vi "Example Grey.vi"() -> ()   [LabVIEW 2020]
uses:
  <vilib>/Utility/sysdir.llb/System Directory Type.ctl
  Sources/_Helpers/Tiff Page Details.ctl
  <vilib>/Analysis/1siggen.llb/Ramp Pattern by Samples.vi
  Sources/TIFF Writer/TIFF Writer.lvclass
  Sources/LV Tiff.lvlib
  Sources/TIFF Reader/TIFF Reader.lvclass
  <vilib>/Analysis/NI_AALBase.lvlib
panel:
  out "DBL":dbl[][](graph)
  out "Read DBL":dbl[][](graph)
  out "U8":u8[][](graph)
  out "Read U8":u8[][](graph)
  out "Read U16":u16[][](graph)
  out "U16":u16[][](graph)
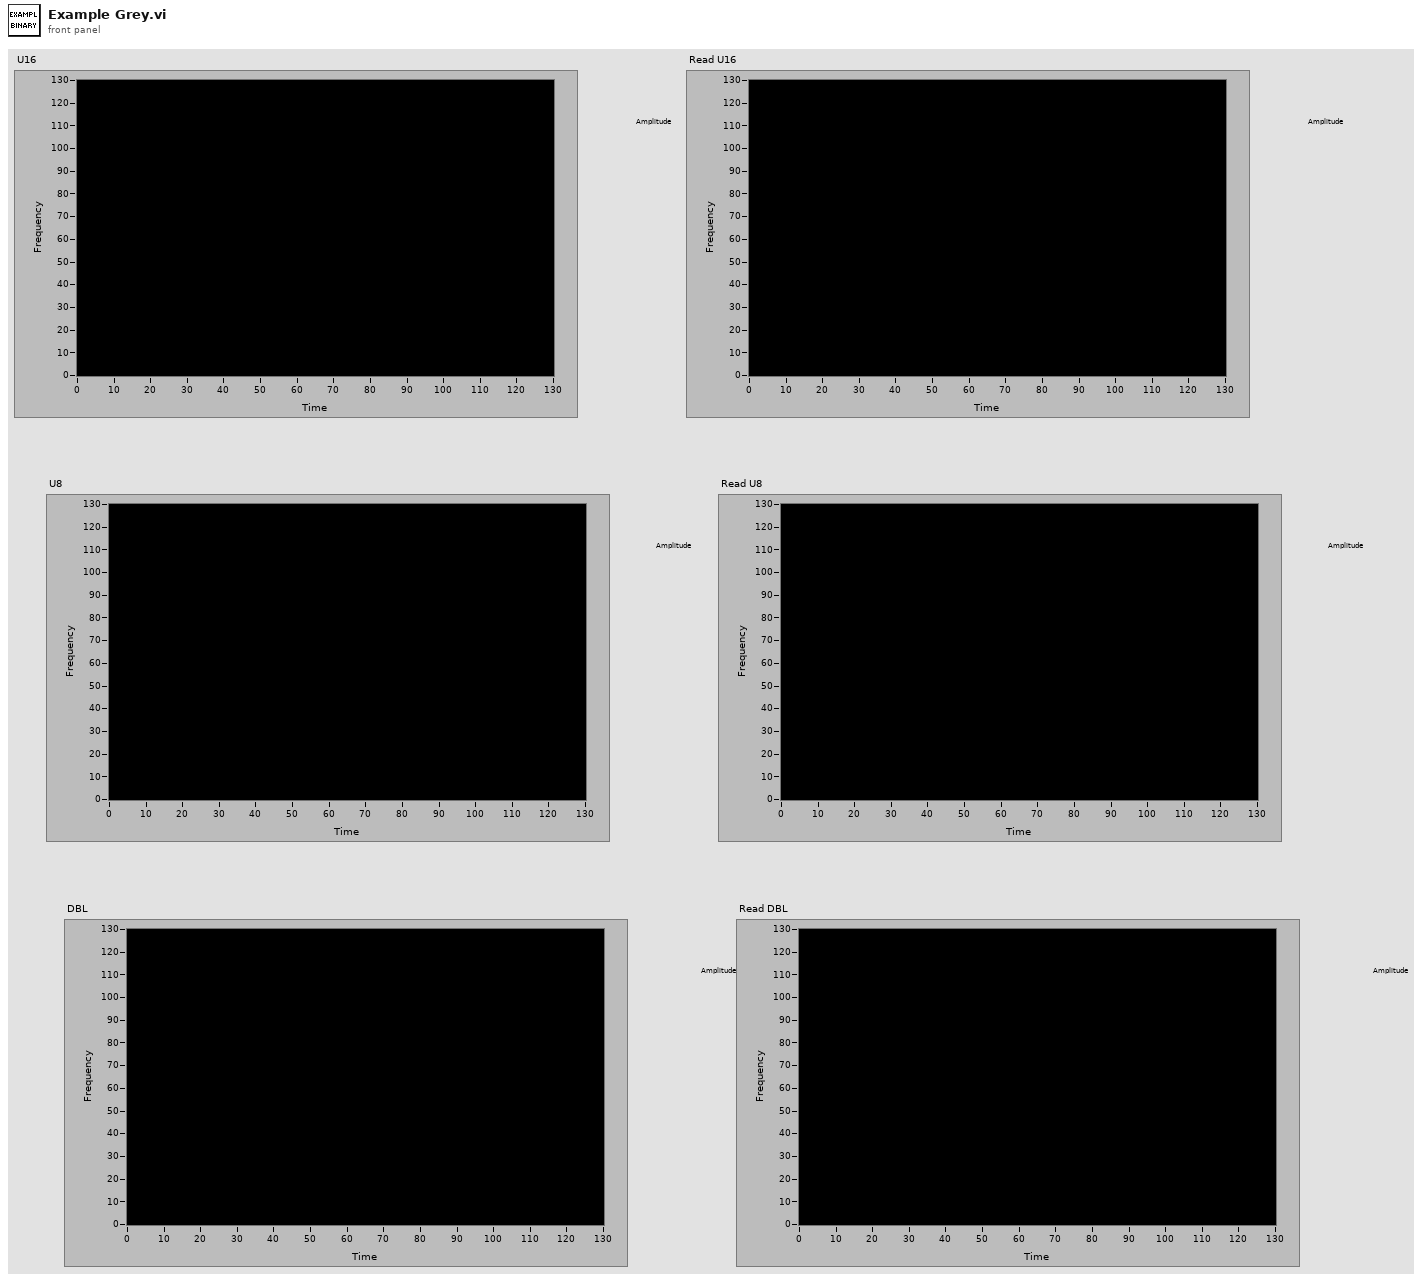
[diagram p1: front panel]
types:
  T1 = typedef "LV Tiff.lvlib/Tiff Page Details.ctl" = cluster{"ImageDescription":string, "XResolution":dbl, "YResolution":dbl, "ResolutionUnit":enum16{"None", "Inch", "Centimeter"}, "PhotometricInterpretation":u16, "Compression":enum16{"None", "Deflate", "JPEG"}, "PageName":string, "DocumentName":string}
  T2 = enum16{"open", "replace", "create", "open or create", "replace or create", "replace or create with confirmation"}
  T3 = typedef "System Directory Type.ctl" = i32
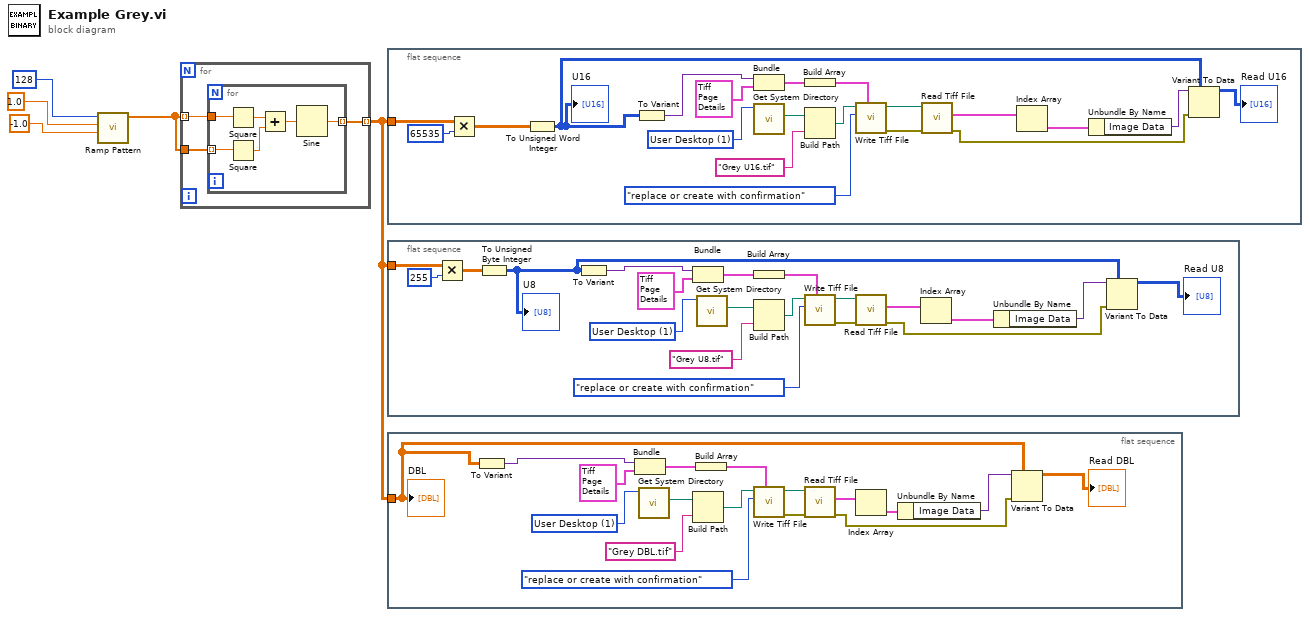
[diagram p0: block diagram]
diagram:
  n1 = call-poly <vilib>:"Ramp Pattern.vi"("start"=-1.0, "end"=1.0, "samples"=128) -> ("Ramp Pattern"=w2:dbl[])  [unwired: 7 in, 1 out]
  n2 = for {
    tunnel: [w8] -> w1 mode=indexing
    tunnel: w2 -> [w7] mode=indexing
    tunnel: w2 -> [w6]
    n3 = for {
      tunnel: [w14] -> w8 mode=indexing
      tunnel: w7 -> [w11]
      tunnel: w6 -> [w10] mode=indexing
      n4 = Square(x=w11) -> (x^2=w12:dbl)
      n5 = Square(x=w10) -> (x^2=w13:dbl)
      n6 = Add(x=w12, y=w13) -> (x+y=w9:dbl)
      n7 = Sine(x=w9) -> (sin(x)=w14:dbl)
    }
  }
  n8 = flat-sequence {
    tunnel: w1 -> [w20]
    frame #0 {
      w17 = T3 1 items=["User Home"=0, "User Desktop"=1, "User Documents"=2, "User Application Data"=3, "User Preferences"=4, "User Temporary"=5, "Public Documents"=6, "Public Application Data"=7, "Public Preferences"=8, "Public Cache"=13, "System Core Libraries"=9, "System Installed Libraries"=10, "Application Files"=11, "Boot Volume Root"=12] ("system directory type")
      n9 = Multiply(x=w20, y=u16 65535) -> (x*y=w33:dbl[][])
      n10 = To Unsigned Word Integer(number=w33) -> (unsigned 16bit integer=w34:u16[][])
      "U16" <- w34
      n11 = To Variant(anything=w34) -> (Variant=w24:variant)
      n12 = Bundle("Variant"=w24, "Details"=T1 {"ImageDescription"="", "XResolution"=0.0, "YResolution"=0.0, "ResolutionUnit"=enum."Inch", "PhotometricInterpretation"=34892, "Compression"=enum."None", "PageName"="", "DocumentName"=""}) -> (w25:cluster{"Variant":variant, "Details":T1})  [unwired: 1 in]
      n13 = call <vilib>:"Get System Directory.vi"("system directory type"=w17) -> ("system directory"=w22:path)  [unwired: 10 in]
      n14 = Build Array(w25) -> (w26:cluster{"Variant":variant, "Details":T1}[])
      n15 = Build Path(base path=w22, name or relative path="Grey U16.tif") -> (appended path=w23:path)
      n16 = call "Write Tiff File.vi"("Pages"=w26, "operation (replace)"=T2."replace or create with confirmation", "Path"=w23) -> ("error out"=w28:errorcluster, "path"=w27:path)  [unwired: 7 in]
      n17 = call "Read Tiff File.vi"("error in (no error)"=w28, "Path"=w27) -> ("error out"=w15:errorcluster, "Pages"=w29:cluster{"Image Data":variant, "Details":T1}[])  [unwired: 6 in, 2 out]
      n18 = Index Array(array=w29) -> (element=w30:cluster{"Image Data":variant, "Details":T1})  [unwired: 1 in]
      n19 = Unbundle By Name(w30) -> ("Image Data"=w31:variant)
      n20 = Variant To Data(error in=w15, type=w34, Variant=w31) -> (data=→"Read U16":u16[][])  [unwired: 1 out]
    }
  }
  n21 = flat-sequence {
    tunnel: w1 -> [w40]
    frame #0 {
      w37 = T3 1 items=["User Home"=0, "User Desktop"=1, "User Documents"=2, "User Application Data"=3, "User Preferences"=4, "User Temporary"=5, "Public Documents"=6, "Public Application Data"=7, "Public Preferences"=8, "Public Cache"=13, "System Core Libraries"=9, "System Installed Libraries"=10, "Application Files"=11, "Boot Volume Root"=12] ("system directory type")
      n22 = Multiply(x=w40, y=u8 255) -> (x*y=w53:dbl[][])
      n23 = To Unsigned Byte Integer(number=w53) -> (unsigned 8bit integer=w54:u8[][])
      "U8" <- w54
      n24 = To Variant(anything=w54) -> (Variant=w44:variant)
      n25 = Bundle("Variant"=w44, "Details"=T1 {"ImageDescription"="", "XResolution"=0.0, "YResolution"=0.0, "ResolutionUnit"=enum."Inch", "PhotometricInterpretation"=34892, "Compression"=enum."None", "PageName"="", "DocumentName"=""}) -> (w45:cluster{"Variant":variant, "Details":T1})  [unwired: 1 in]
      n26 = call <vilib>:"Get System Directory.vi"("system directory type"=w37) -> ("system directory"=w42:path)  [unwired: 10 in]
      n27 = Build Array(w45) -> (w46:cluster{"Variant":variant, "Details":T1}[])
      n28 = Build Path(base path=w42, name or relative path="Grey U8.tif") -> (appended path=w43:path)
      n29 = call "Write Tiff File.vi"("Pages"=w46, "operation (replace)"=T2."replace or create with confirmation", "Path"=w43) -> ("error out"=w48:errorcluster, "path"=w47:path)  [unwired: 7 in]
      n30 = call "Read Tiff File.vi"("error in (no error)"=w48, "Path"=w47) -> ("error out"=w35:errorcluster, "Pages"=w49:cluster{"Image Data":variant, "Details":T1}[])  [unwired: 6 in, 2 out]
      n31 = Index Array(array=w49) -> (element=w50:cluster{"Image Data":variant, "Details":T1})  [unwired: 1 in]
      n32 = Unbundle By Name(w50) -> ("Image Data"=w51:variant)
      n33 = Variant To Data(error in=w35, type=w54, Variant=w51) -> (data=→"Read U8":u8[][])  [unwired: 1 out]
    }
  }
  n34 = flat-sequence {
    tunnel: w1 -> [w56]
    frame #0 {
      w58 = T3 1 items=["User Home"=0, "User Desktop"=1, "User Documents"=2, "User Application Data"=3, "User Preferences"=4, "User Temporary"=5, "Public Documents"=6, "Public Application Data"=7, "Public Preferences"=8, "Public Cache"=13, "System Core Libraries"=9, "System Installed Libraries"=10, "Application Files"=11, "Boot Volume Root"=12] ("system directory type")
      n35 = To Variant(anything=w56) -> (Variant=w63:variant)
      n36 = Bundle("Variant"=w63, "Details"=T1 {"ImageDescription"="", "XResolution"=0.0, "YResolution"=0.0, "ResolutionUnit"=enum."Inch", "PhotometricInterpretation"=34892, "Compression"=enum."None", "PageName"="", "DocumentName"=""}) -> (w64:cluster{"Variant":variant, "Details":T1})  [unwired: 1 in]
      n37 = call <vilib>:"Get System Directory.vi"("system directory type"=w58) -> ("system directory"=w61:path)  [unwired: 10 in]
      n38 = Build Path(base path=w61, name or relative path="Grey DBL.tif") -> (appended path=w62:path)
      n39 = Build Array(w64) -> (w65:cluster{"Variant":variant, "Details":T1}[])
      n40 = call "Write Tiff File.vi"("Pages"=w65, "operation (replace)"=T2."replace or create with confirmation", "Path"=w62) -> ("error out"=w67:errorcluster, "path"=w66:path)  [unwired: 7 in]
      n41 = call "Read Tiff File.vi"("error in (no error)"=w67, "Path"=w66) -> ("error out"=w55:errorcluster, "Pages"=w68:cluster{"Image Data":variant, "Details":T1}[])  [unwired: 6 in, 2 out]
      n42 = Index Array(array=w68) -> (element=w69:cluster{"Image Data":variant, "Details":T1})  [unwired: 1 in]
      n43 = Unbundle By Name(w69) -> ("Image Data"=w70:variant)
      n44 = Variant To Data(error in=w55, type=w56, Variant=w70) -> (data=→"Read DBL":dbl[][])  [unwired: 1 out]
      "DBL" <- w56
    }
  }
